vi "hexStrConv.vi"(0 "Input ASCII Hex String":string, 1 "error in (no error)":errorcluster) -> (2 "Output Non Printable HEX String":string, 3 "Checksum HEX String":string, 4 "error out":errorcluster)   [LabVIEW 2019]
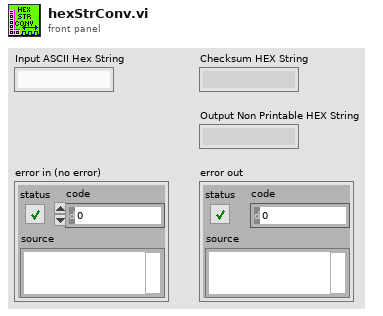
[diagram p1: front panel]
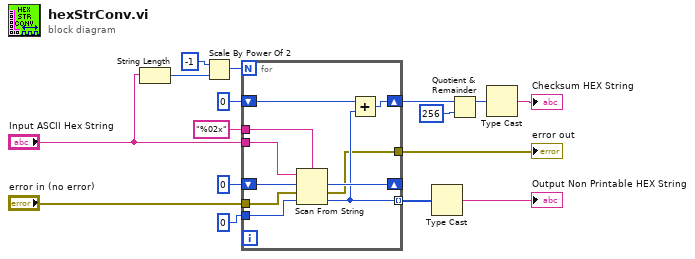
[diagram p0: block diagram]
diagram:
  n1 = String Length(string="Input ASCII Hex String") -> (length=w2:i32)
  n2 = Scale By Power Of 2(n=i16 -1, x=w2) -> (x*2^n=w4:i32)
  n3 = for {
    N: w4 -> [_]
    tunnel: "Input ASCII Hex String" -> [w26]
    tunnel: "%02x" -> [w25]
    shift-right: [w24] -> _
    shift-left: u32 0 -> [w23]
    tunnel: u8 0 -> [w22]
    tunnel: [w21] -> w7 mode=indexing
    shift-right: [w20] -> w8
    shift-left: u8 0 -> [w19]
    tunnel: "error in (no error)" -> [w18]
    tunnel: [w17] -> w16
    n4 = Scan From String(format string=w25, input string=w26, initial scan location=w23, error in=w18, default 1=w22) -> (offset past scan=w24:u32, error out=w17:errorcluster, output 1=w21:u8)  [unwired: 1 out]
    n5 = Add(x=w19, y=w21) -> (x+y=w20:u8)
  }
  "error out" <- w16
  n6 = Type Cast(x=w7) -> (*(type *) &x=→"Output Non Printable HEX String":string)  [unwired: 1 in]
  n7 = Quotient & Remainder(x=w8, y=u16 256) -> (x-y*floor(x/y)=w13:u16)  [unwired: 1 out]
  n8 = Type Cast(x=w13) -> (*(type *) &x=→"Checksum HEX String":string)  [unwired: 1 in]
